vi "F Dwf Analog In Status.vi"(8 "error in (no error)":errorcluster, 9 "psts":string, 10 "fReadData":i32, 11 "hdwf":i32) -> (0 "error out":errorcluster, 1 "psts out":string, 3 "function return":i32)   [LabVIEW 2021, in "Olasdwf.lvlib"]
doc: "DWFAPI int FDwfAnalogInStatus(HDWF hdwf, int fReadData, DwfState *psts);"
uses:
  Olasdwf.lvlib
  Windows/System32/dwf.dll
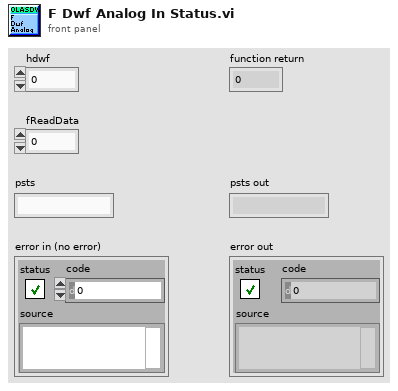
[diagram p1: front panel]
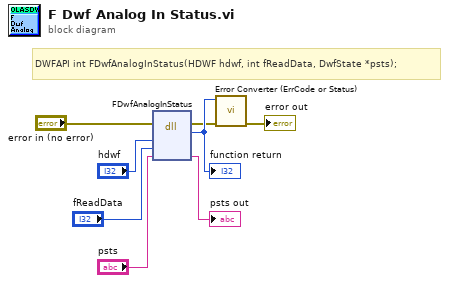
[diagram p0: block diagram]
diagram:
  # "DWFAPI int FDwfAnalogInStatus(HDWF hdwf, int fReadData, DwfState *psts);"
  n1 = dll-call lib="/Windows/System32/dwf.*" fn="FDwfAnalogInStatus"(error in="error in (no error)", "hdwf"="hdwf", "fReadData"="fReadData", "psts"="psts") -> (error out=w2:errorcluster, w8:i32, "psts"=→"psts out":string)  [unwired: 4 in, 1 out]
  "function return" <- w8
  n2 = call "Error Converter (ErrCode or Status).vi"("error in (no error)"=w2, "error code"=w8) -> ("error out"=→"error out":errorcluster)  [unwired: 9 in]
